vi "event_subscriber.vi"() -> ()   [LabVIEW 2016]
uses:
  ts_sallv_exa/SALLV_EXA.lvlib
panel:
  out "State":T1(ring)
  out "Heartbean?":bool=TRUE
  out "Count":i32
  out "Stop 2":bool=TRUE
  out "Stop":bool=TRUE
  in  "stop":bool
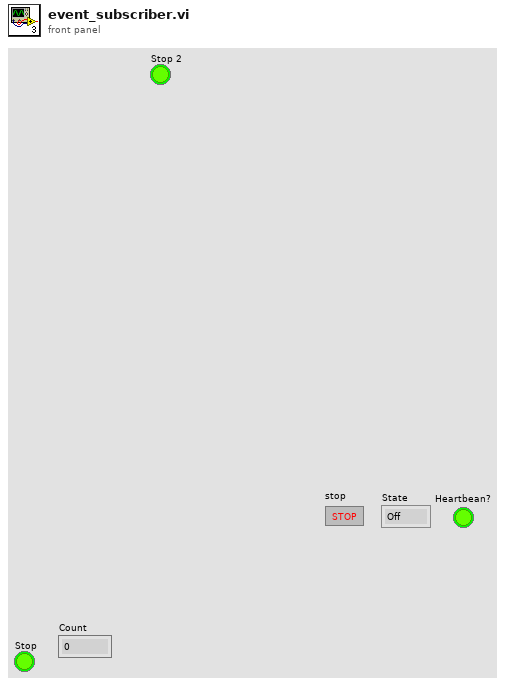
[diagram p1: front panel]
types:
  T1 = enum16{"Off", "Standby", "Enable", "Disable", "Fault"}
  T2 = typedef "SALLV_EXA.lvlib/logevent_SummaryState.ctl" = cluster{"SummaryStateValue":i32, "priority":i32}
  T3 = typedef "SALLV_EXA.lvlib/logevent_Heartbeat.ctl" = cluster{"Heartbeat":bool, "priority":i32}
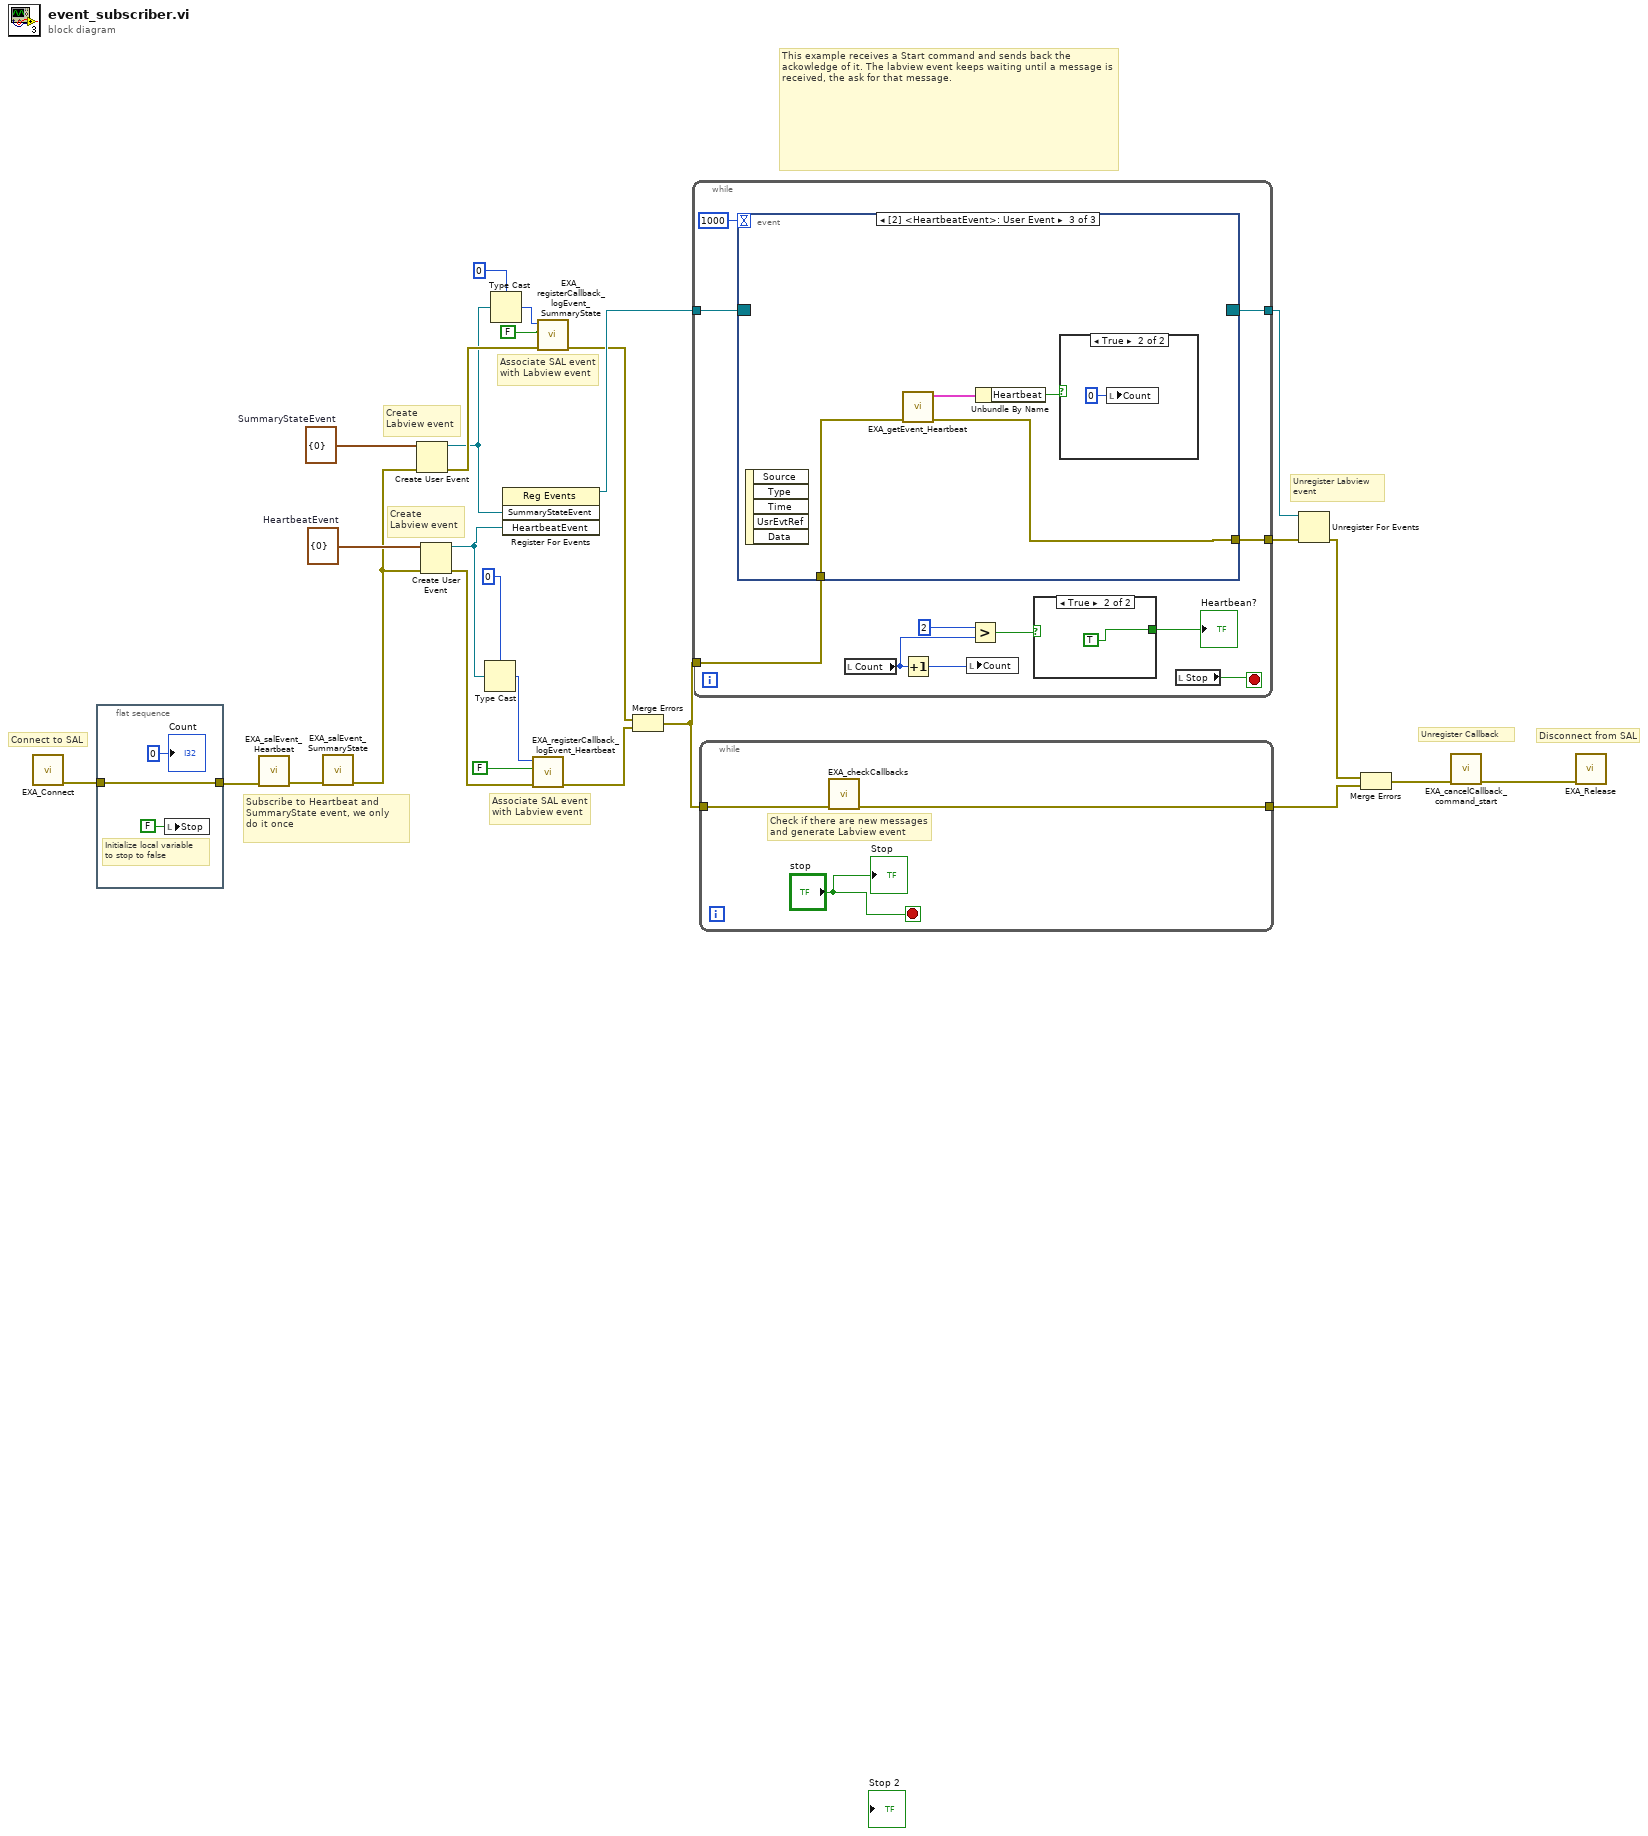
[diagram p0: block diagram]
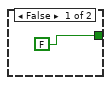
[diagram p2: hidden frame]
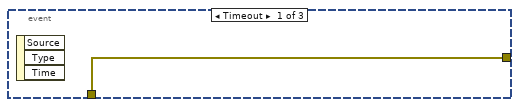
[diagram p3: hidden frame]
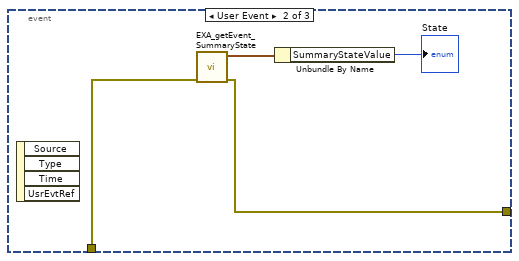
[diagram p4: hidden frame]
diagram:
  w12 = cluster{"Data":i32} {"Data"=0}  # SummaryStateEvent
  w25 = cluster{"Data":i32} {"Data"=0}  # HeartbeatEvent
  # "Create Labview event"
  # "Associate SAL event\nwith Labview event"
  # "This example receives a Start command and sends back the ackowledge of it. The labview event keeps waiting until a message is received, the ask for that message."
  # "Unregister Labview\nevent"
  # "Create Labview event"
  # "Associate SAL event\nwith Labview event"
  # "Unregister Callback"
  # "Subscribe to Heartbeat and SummaryState event, we only\ndo it once"
  # "Disconnect from SAL"
  # "Connect to SAL"
  n1 = call "EXA_Connect.vi"() -> ("error out"=w26:errorcluster)  [unwired: 10 in, 1 out]
  n2 = flat-sequence {
    tunnel: w26 -> [w28]
    tunnel: [w28] -> w15
    frame #0 {
      # "Initialize local variable \nto stop to false"
      n3 = local write "Stop"(FALSE ("Stop")) -> ()
      "Count" <- 0 ("Count")
    }
  }
  n4 = call "EXA_salEvent_Heartbeat.vi"("error in (no error)"=w15) -> ("error out"=w16:errorcluster)  [unwired: 9 in, 1 out]
  n5 = call "EXA_salEvent_SummaryState.vi"("error in (no error)"=w16) -> ("error out"=w10:errorcluster)  [unwired: 9 in, 1 out]
  n6 = Create User Event(user event datatype=w12, error in=w10) -> (user event=w4:refnum<user-event>, error out=w7:errorcluster)
  n7 = Create User Event(user event datatype=w25, error in=w10) -> (user event=w11:refnum<user-event>, error out=w8:errorcluster)
  n8 = Type Cast(type=0 ("handle"), x=w11) -> (*(type *) &x=w13:i32)
  n9 = Type Cast(type=0 ("handle"), x=w4) -> (*(type *) &x=w5:i32)
  n10 = register-events(w4, w11) -> (reference out=w23:refnum<event-registration>)  [unwired: 2 in, 1 out]
  n11 = call "EXA_registerCallback_logEvent_Heartbeat.vi"("error in (no error)"=w8, "skipOld"=FALSE, "handle"=w13) -> ("error out"=w2:errorcluster)  [unwired: 7 in, 1 out]
  n12 = call "EXA_registerCallback_logEvent_SummaryState.vi"("error in (no error)"=w7, "skipOld"=FALSE, "handle"=w5) -> ("error out"=w1:errorcluster)  [unwired: 7 in, 1 out]
  n13 = Merge Errors(w1, w2) -> (w3:errorcluster)
  n14 = while {
    tunnel: w23 -> [w38]
    tunnel: w3 -> [w37]
    tunnel: [w36] -> w19
    tunnel: [w35] -> w18
    stop <- w40 stop-if-true
    n15 = event shown="[2] <HeartbeatEvent>: User Event" {
      selector: w38 -> [_ _ _]
      dyn-events: [_ _ _] -> w35
      timeout: 1000 -> [_ _ _]
      tunnel: w37 -> [w43 w47 w51]
      tunnel: [w43 w46 w48] -> w36
      event Timeout {
        n16 = event-data() -> ()  [unwired: 1 in, 3 out]
      }
      event User Event {
        n17 = event-data() -> ()  [unwired: 1 in, 4 out]
        n18 = call "EXA_getEvent_SummaryState.vi"("error in (no error)"=w47) -> ("error out"=w46:errorcluster, "logevent_SummaryState_Ctl out"=w45:T2)  [unwired: 8 in, 1 out]
        n19 = Unbundle By Name(w45) -> ("SummaryStateValue"=→"State":i32)
      }
      event User Event {
        n20 = event-data() -> ()  [unwired: 1 in, 5 out]
        n21 = call "EXA_getEvent_Heartbeat.vi"("error in (no error)"=w51) -> ("error out"=w48:errorcluster, "logevent_Heartbeat_Ctl out"=w50:T3)  [unwired: 8 in, 1 out]
        n22 = Unbundle By Name(w50) -> ("Heartbeat"=w49:bool)
        n23 = case shown="True" w49 {
          frame False {
          }
          frame True {
            n24 = local write "Count"(0 ("Count")) -> ()
          }
        }
      }
    }
    n25 = local read "Count"() -> (w30:i32)
    n26 = Increment(x=w30) -> (x+1=w31:i32)
    n27 = local write "Count"(w31) -> ()
    n28 = Greater?(x=2 ("y"), y=w30) -> (0:w33:bool)
    n29 = case shown="True" w33 {
      tunnel: [FALSE TRUE] -> w34
      frame False {
      }
      frame True {
      }
    }
    "Heartbean?" <- w34
    n30 = local read "Stop"() -> (w40:bool)
  }
  n31 = while {
    tunnel: w3 -> [w54]
    tunnel: [w53] -> w21
    stop <- "stop" stop-if-true
    # "Check if there are new messages \nand generate Labview event"
    n32 = call "EXA_checkCallbacks.vi"("error in (no error)"=w54) -> ("error out"=w53:errorcluster)  [unwired: 10 in]
    "Stop" <- "stop"
  }
  n33 = Unregister For Events(event registration refnum=w18, error in=w19) -> (error out=w17:errorcluster)
  n34 = Merge Errors(w17, w21) -> (w20:errorcluster)
  n35 = call "EXA_cancelCallback_command_start.vi"("error in (no error)"=w20) -> ("error out"=w22:errorcluster)  [unwired: 9 in, 1 out]
  n36 = call "EXA_Release.vi"("error in (no error)"=w22) -> ()  [unwired: 9 in, 2 out]
